vi "Generate Alarm Appeared Log Entry.vi"(11 "Alarm":T1) -> (3 "Log Entry":string)   [LabVIEW 2015, in "Alarm Handler Actor.lvclass"]
uses:
  Alarm Handler Actor.lvclass
  Active Alarm.ctl
  Alarm Details.ctl
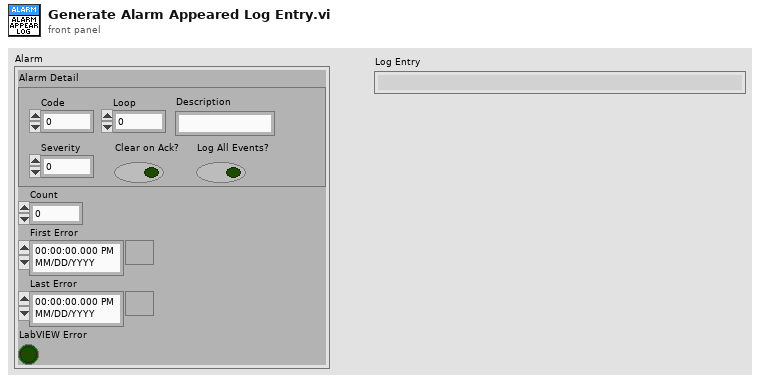
[diagram p1: front panel]
types:
  T1 = typedef "Alarm Handler Actor.lvclass/Active Alarm.ctl" = cluster{"Alarm Detail":T2, "Count":i32, "First Error":timestamp, "Last Error":timestamp, "LabVIEW Error":bool}
  T2 = typedef "Alarm Handler Actor.lvclass/Alarm Details.ctl" = cluster{"Code":i32, "Loop":i32, "Description":string, "Severity":i32, "Clear on Ack?":bool, "Log All Events?":bool}
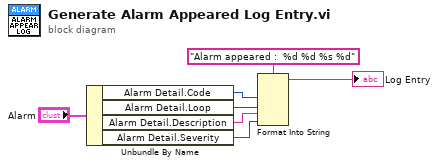
[diagram p0: block diagram]
diagram:
  n1 = Unbundle By Name("Alarm") -> ("Alarm Detail.Code"=w4:i32, "Alarm Detail.Loop"=w5:i32, "Alarm Detail.Description"=w6:string, "Alarm Detail.Severity"=w7:i32)
  n2 = Format Into String(format string="Alarm appeared :  %d %d %s %d", w4, w5, w6, w7) -> (resulting string=→"Log Entry":string)  [unwired: 2 in, 1 out]
